vi "Command-Line.vi"() -> ()   [LabVIEW 2014]
panel:
  out "Standard Output":string
  in  "Command Line":string
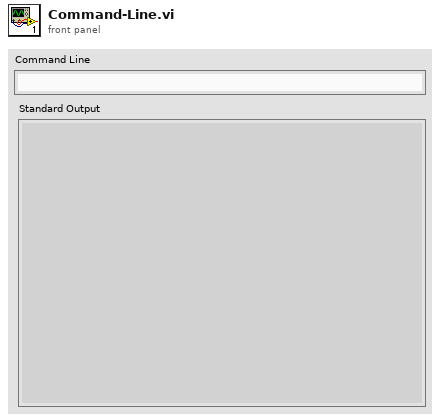
[diagram p1: front panel]
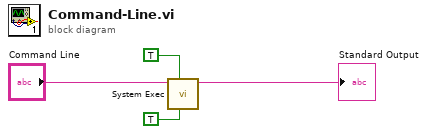
[diagram p0: block diagram]
diagram:
  n1 = call <vilib>:"System Exec.vi"("run minimized? (F)"=TRUE, "wait until completion? (T)"=TRUE, "command line"="Command Line") -> ("standard output"=→"Standard Output":string)  [unwired: 5 in, 3 out]
